vi "CamIndex.vi"(6 "index":i32, 8 "error in (no error)":errorcluster, 11 "MagAnalysis_Online in":refnum<class "MagAnalysis_Online.lvclass">) -> (0 "error out":errorcluster, 1 "Cam Cluster out 2":T5={"incident ANGLE COMPENSATION"=[], "field of view /pixel"=0.0, "dp/B [MeV/C/B]"=[], "charge compensation"=[], "Momentum [MeV/C]"=[], "B [T]"=1.0, "energyDependence Input"=[], "pixel angle (y)"=[], "dp [MeV/C/] "=[], "angle 2Dfor spectrumj"=[], "dp [MeV/C] 2D"=[], "charge compensation 2D"=[], "Screen&Camera 2"={"Screen Orientation"="Regular", "Screen angle"="Flat", "Lens"=enum."FL1-f8x08", "Calibration (mm/pix)"=1.0}, "ROI info"={"npix-X"=0, "npix-Y"=0, "Left [pix]"=0.0, "Top [pix]"=0.0}, "Y 2D full angle"=[]}, 2 "spec cluster":T4, 3 "z":dbl[][](array[numeric]), 7 "time":u32)   [LabVIEW 2011, in "MagAnalysis_Online.lvclass"]
uses:
  MagAnalysis_Online.lvclass
  calib_Sub_Typdef.ctl
  ScreenCam2_TypDEf.ctl
  CamAndObj_TypDEf.ctl
  ROIInfo_TypDef.ctl
  specCluster_Typdef.ctl
  reshapeINfo_TypDef.ctl
  emptyArray_TYpDEf.ctl
  emptyArrayCamX_TypDef.ctl
  specClustercommandTypdef.ctl
  MagAnalysis_Online.lvclass/MagAnalysis_Online.ctl
  reshapeArrayCommand_TypDEf.ctl
panel:
  in  "reshapeInfo":T1
  out "time:spec":u32
  out "time:cliab":u32
  out "FGV":u32
  out "time: AllProc":u32
  out "time":u32
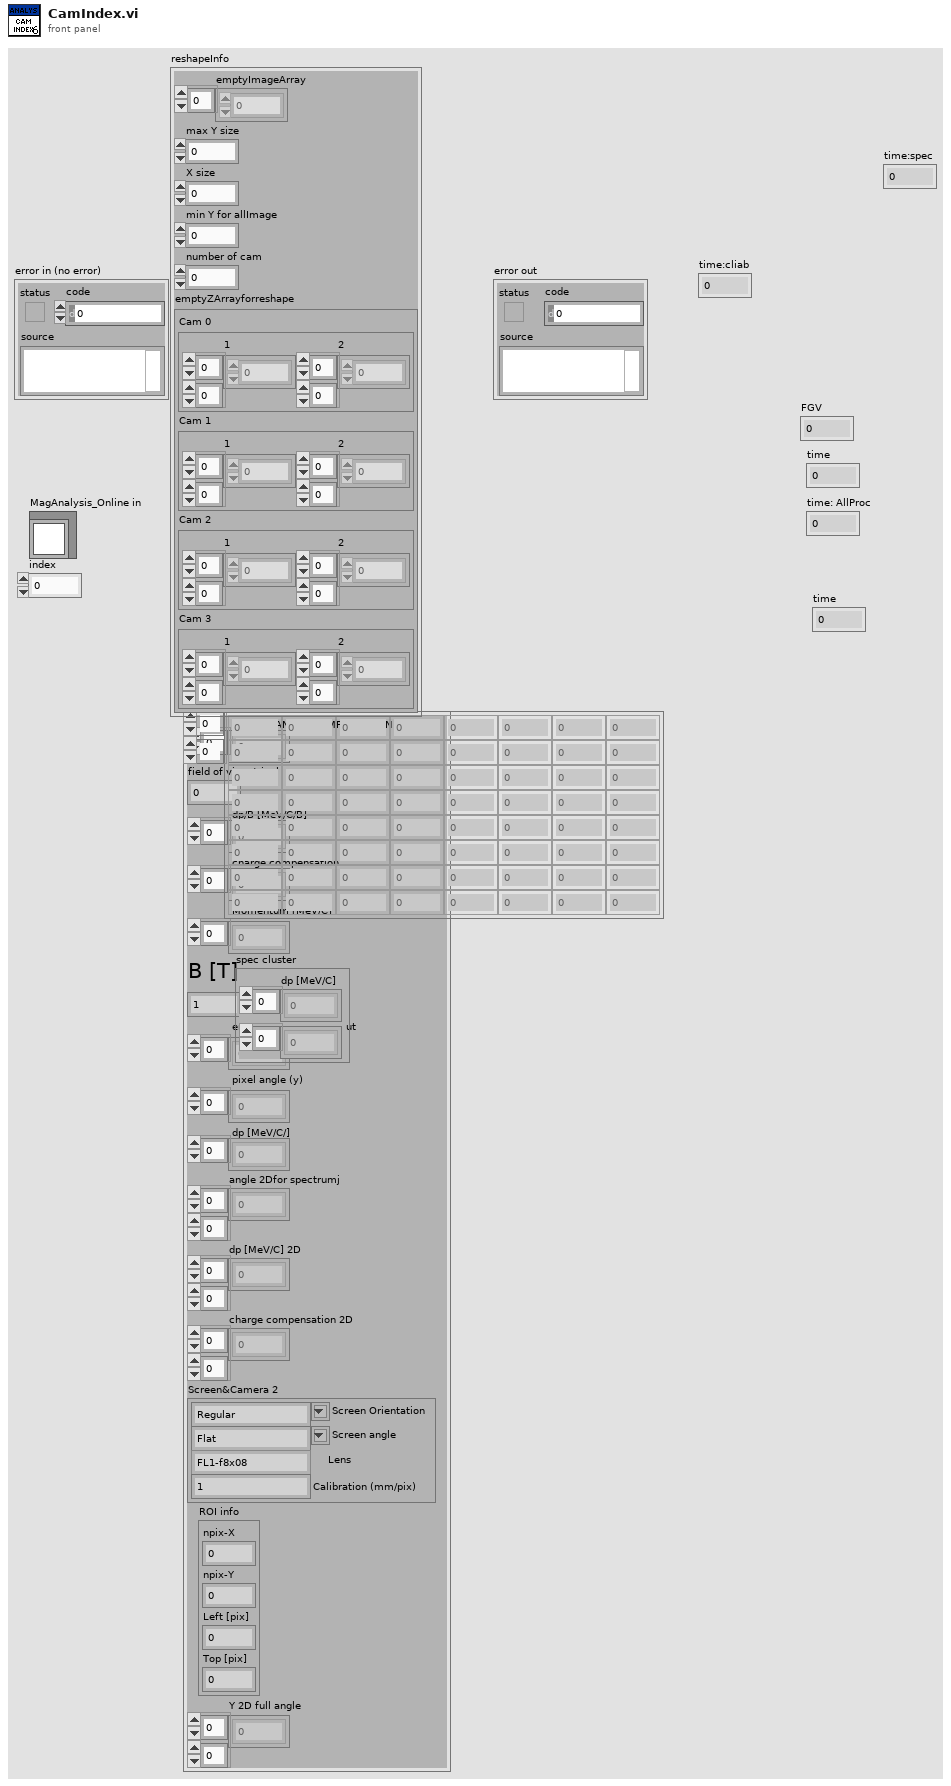
[diagram p1: front panel]
types:
  T1 = typedef "reshapeINfo_TypDef.ctl" = cluster{"emptyImageArray":dbl[], "max Y size":i32, "X size":i32, "min Y for allImage":dbl, "number of cam":i32, "emptyZArrayforreshape":T2}
  T2 = typedef "emptyArray_TYpDEf.ctl" = cluster{"Cam 0":T3, "Cam 1":T3, "Cam 2":T3, "Cam 3":T3}
  T3 = typedef "emptyArrayCamX_TypDef.ctl" = cluster{"1":dbl[][], "2":dbl[][]}
  T4 = typedef "specCluster_Typdef.ctl" = cluster{"dp [MeV/C]":dbl[], dbl[]}
  T5 = typedef "calib_Sub_Typdef.ctl" = cluster{"incident ANGLE COMPENSATION":dbl[], "field of view /pixel":dbl, "dp/B [MeV/C/B]":dbl[], "charge compensation":dbl[], "Momentum [MeV/C]":dbl[], "B [T]":dbl, "energyDependence Input":dbl[], "pixel angle (y)":dbl[], "dp [MeV/C/] ":dbl[], "angle 2Dfor spectrumj":dbl[][], "dp [MeV/C] 2D":dbl[][], "charge compensation 2D":dbl[][], "Screen&Camera 2":T6, "ROI info":T8, "Y 2D full angle":dbl[][]}
  T6 = typedef "ScreenCam2_TypDEf.ctl" = cluster{"Screen Orientation":string, "Screen angle":string, "Lens":T7, "Calibration (mm/pix)":dbl}
  T7 = typedef "CamAndObj_TypDEf.ctl" = enum16{"FL1-f8x08", "FL1-f8x06", "FL1-f8", "ch300-f50", "FL2G-f8", "FL3M14-f8", "FL3M14-f8x08", "FL3M14-f8x08(2x2)"}
  T8 = typedef "ROIInfo_TypDef.ctl" = cluster{"npix-X":i32, "npix-Y":i32, "Left [pix]":dbl, "Top [pix]":dbl}
  T9 = typedef "specClustercommandTypdef.ctl" = enum16{"init", "addCluster", "read"}
  T10 = typedef "reshapeArrayCommand_TypDEf.ctl" = enum16{"init array", "addImage", "read", "init resolution"}
  T11 = typedef "MagAnalysis_Online.lvclass/analysis_data_typdef.ctl" = cluster{"cam0":T12, "cam1":T12, "cam2":T12, "cam3":T12}
  T12 = typedef "IMAQ Image.ctl" = refnum<image>
  T13 = typedef "bgImages_tyudef.ctl" = cluster{"cam 0":T12, "cam 1":T12, "cam 2":T12, "cam 3":T12}
  T14 = typedef "CamSettings_Typdef.ctl" = cluster{"Cam 0":T15, "Cam 1":T15, "Cam 2":T15, "Cam 3":T15}
  T15 = typedef "CamSettingSUB_TypDEf.ctl" = cluster{"position":dbl, "Field of view":dbl, "start":dbl, "end":dbl, "center":dbl, "Lens":T7, "Forward":T16, "Spec_Calib_file 2":path, "map":path, "y size":i32}
  T16 = typedef "OnOffTypeDef.ctl" = enum16{"off", "on"}
  T17 = cluster{"S 0":i32[][], "S 1":i32[][], "S 2":i32[][], "S 3":i32[][]}
  T18 = typedef "Calib_Typdef.ctl" = cluster{"cam 0":T5, "cam 1":T5, "cam 2":T5, "cam 3":T5}
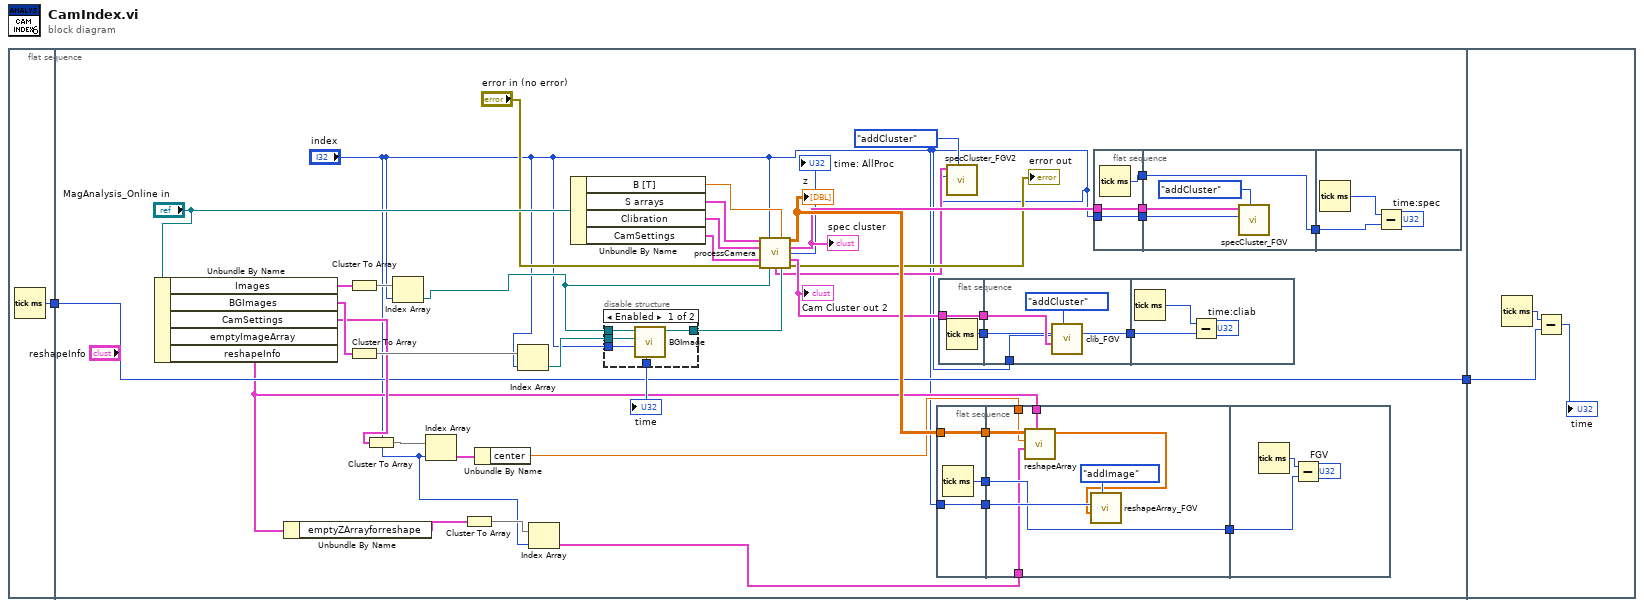
[diagram p0: block diagram]
diagram:
  n1 = flat-sequence {
    tunnel: [w3] -> w2
    tunnel: w2 -> [w26]
    tunnel: [w26] -> w1
    tunnel: w1 -> [w85]
    frame #0 {
      n2 = Tick Count (ms)() -> (millisecond timer value=w3:u32)
    }
    frame #1 {
      n3 = Unbundle By Name("MagAnalysis_Online in") -> ("Images"=w35:T11, "BGImages"=w34:T13, "CamSettings"=w33:T14, "reshapeInfo"=w13:T1)  [unwired: 1 out]
      n4 = Unbundle By Name(w13) -> ("emptyZArrayforreshape"=w12:T2)
      n5 = Cluster To Array(cluster=w35) -> (array=w43:T12[])
      n6 = Cluster To Array(cluster=w34) -> (array=w44:T12[])
      n7 = Cluster To Array(cluster=w33) -> (array=w32:T15[])
      n8 = Index Array(array=w43, index="index") -> (element=w38:T12)
      n9 = Index Array(array=w32, index="index") -> (element=w31:T15)
      n10 = Cluster To Array(cluster=w12) -> (array=w11:T3[])
      n11 = Unbundle By Name(w31) -> ("center"=w9:dbl)
      n12 = Index Array(array=w44, index="index") -> (element=w45:T12)
      n13 = Index Array(array=w11, index="index") -> (element=w10:T3)
      n14 = Unbundle By Name("MagAnalysis_Online in") -> ("B [T]"=w37:dbl, "S arrays"=w40:T17, "Clibration"=w41:T18, "CamSettings"=w42:T14)
      n15 = disable-structure shown="Enabled" {
        disable-tunnel: w45 -> [w50 w51]
        disable-tunnel: [w49 w51] -> w39
        disable-tunnel: w38 -> [w48 _]
        disable-tunnel: "index" -> [w47 _]
        disable-tunnel: [w46 _] -> w27
        frame Enabled {
          n16 = call "BGImage.vi"("index"=w47, "BG"=w50, "Image"=w48) -> ("Refnum out"=w49:T12, "time"=w46:u32)  [unwired: 7 in]
        }
        frame Disabled {
        }
      }
      "time" <- w27
      n17 = call "processCamera.vi"("S arrays"=w40, "index"="index", "B [T]"=w37, "Clibration"=w41, "CamSettings"=w42, "error in (no error)"="error in (no error)", "image in"=w38, "bg in"=w39) -> ("z"=w30:dbl[][], "spec cluster"=w29:cluster{"dp [MeV/C]":dbl[], dbl[]}, "time: AllProc"=→"time: AllProc":u32, "Cam Cluster out 2"=w28:T5, "Sum Y"=w6:cluster{"Ramp Pattern":dbl[], dbl[]}, "error out"=→"error out":errorcluster)  [unwired: 2 in]
      "Cam Cluster out 2" <- w28
      "spec cluster" <- w29
      "z" <- w30
      n18 = flat-sequence {
        tunnel: "index" -> [w72]
        tunnel: w30 -> [w73]
        tunnel: [w73] -> w24
        tunnel: [w72] -> w23
        tunnel: [w71] -> w22
        tunnel: w24 -> [w81]
        tunnel: w23 -> [w80]
        tunnel: w22 -> [w78]
        tunnel: [w78] -> w21
        tunnel: w13 -> [w76]
        tunnel: w10 -> [w75]
        tunnel: w9 -> [w74]
        tunnel: w21 -> [w82]
        frame #0 {
          n19 = Tick Count (ms)() -> (millisecond timer value=w71:u32)
        }
        frame #1 {
          n20 = call "reshapeArray.vi"("reshapeInfo"=w76, "element"=w75, "center"=w74, "z"=w81) -> ("reshaped array"=w77:dbl[])  [unwired: 7 in]
          n21 = call "reshapeArray_FGV.vi"("command"=reshapeArrayCommand_TypDEf."addImage", "reshapedArray CamX"=w77, "index"=w80) -> ()  [unwired: 7 in, 2 out]
        }
        frame #2 {
          n22 = Tick Count (ms)() -> (millisecond timer value=w83:u32)
          n23 = Subtract(x=w83, y=w82) -> (x-y=→"FGV":u32)
        }
      }
      n24 = flat-sequence {
        tunnel: w28 -> [w63]
        tunnel: [w63] -> w20
        tunnel: [w62] -> w19
        tunnel: "index" -> [w66]
        tunnel: w20 -> [w67]
        tunnel: w19 -> [w64]
        tunnel: [w64] -> w18
        tunnel: w18 -> [w68]
        frame #0 {
          n25 = Tick Count (ms)() -> (millisecond timer value=w62:u32)
        }
        frame #1 {
          n26 = call "clib_FGV.vi"("command"=specClustercommandTypdef."addCluster", "Cam Cluster out 2"=w67, "index"=w66) -> ()  [unwired: 7 in, 2 out]
        }
        frame #2 {
          n27 = Tick Count (ms)() -> (millisecond timer value=w69:u32)
          n28 = Subtract(x=w69, y=w68) -> (x-y=→"time:cliab":u32)
        }
      }
      n29 = call "specCluster_FGV2.vi"("command"=specClustercommandTypdef."addCluster", "index"="index", "spec cluster"=w6) -> ()  [unwired: 7 in, 2 out]
      n30 = flat-sequence {
        tunnel: "index" -> [w53]
        tunnel: w29 -> [w54]
        tunnel: [w54] -> w17
        tunnel: [w53] -> w16
        tunnel: [w52] -> w14
        tunnel: w17 -> [w58]
        tunnel: w16 -> [w57]
        tunnel: [w55] -> w15
        tunnel: w14 -> [w55]
        tunnel: w15 -> [w59]
        frame #0 {
          n31 = Tick Count (ms)() -> (millisecond timer value=w52:u32)
        }
        frame #1 {
          n32 = call "specCluster_FGV.vi"("command"=specClustercommandTypdef."addCluster", "index"=w57, "spec cluster"=w58) -> ()  [unwired: 7 in, 2 out]
        }
        frame #2 {
          n33 = Tick Count (ms)() -> (millisecond timer value=w61:u32)
          n34 = Subtract(x=w61, y=w59) -> (x-y=→"time:spec":u32)
        }
      }
    }
    frame #2 {
      n35 = Tick Count (ms)() -> (millisecond timer value=w87:u32)
      n36 = Subtract(x=w87, y=w85) -> (x-y=→"time":u32)
    }
  }
